vi "Update Control.vi"(8 "error in (no error)":errorcluster, 9 "Default Value Map":variant, 10 "Value":variant, 11 "Control Ref":refnum<vi>) -> (0 "error out":errorcluster, 1 "Label Text":string, 2 "Value":variant, 3 "Control Ref":refnum<vi>)   [LabVIEW 2019, in "User Interface.lvlib"]
doc: "Handles updating fill for knob and slide controls. Will also update output type as necessary (see note on block diagram)."
uses:
  User Interface.lvlib
  <vilib>/Utility/Data Type/NI_Data Type.lvlib
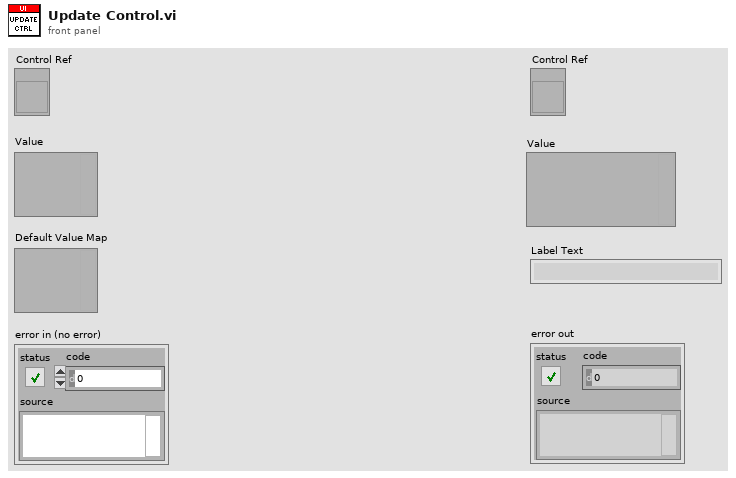
[diagram p1: front panel]
types:
  T1 = typedef "NI_Data Type.lvlib/Data Type.ctl" = enum8{"Invalid Type", "Void", "I8", "I16", "I32", "I64", "U8", "U16", "U32", "U64", "Single Float", "Double Float", "Extended Float", "Single Complex", "Double Complex", "Extended Complex", "Enum U8", "Enum U16", "Enum U32", "Enum U64", "Single Float With Unit", "Double Float With Unit", "Extended Float With Unit", "Single Complex with Unit", "Double Complex with Unit", "Extended Complex with Unit", "Boolean", "String", "Path", "Picture", "Tag", "Array", "Cluster", "Variant", "LV Variant", "Waveform", "Timestamp", "Digital Waveform", "Digital Data", "ExpressData", "Refnum", "External Data", "VI", "Poly VI", "LabVIEW Class Instance", "Fixed Point", "Set Collection", "Map Collection"}
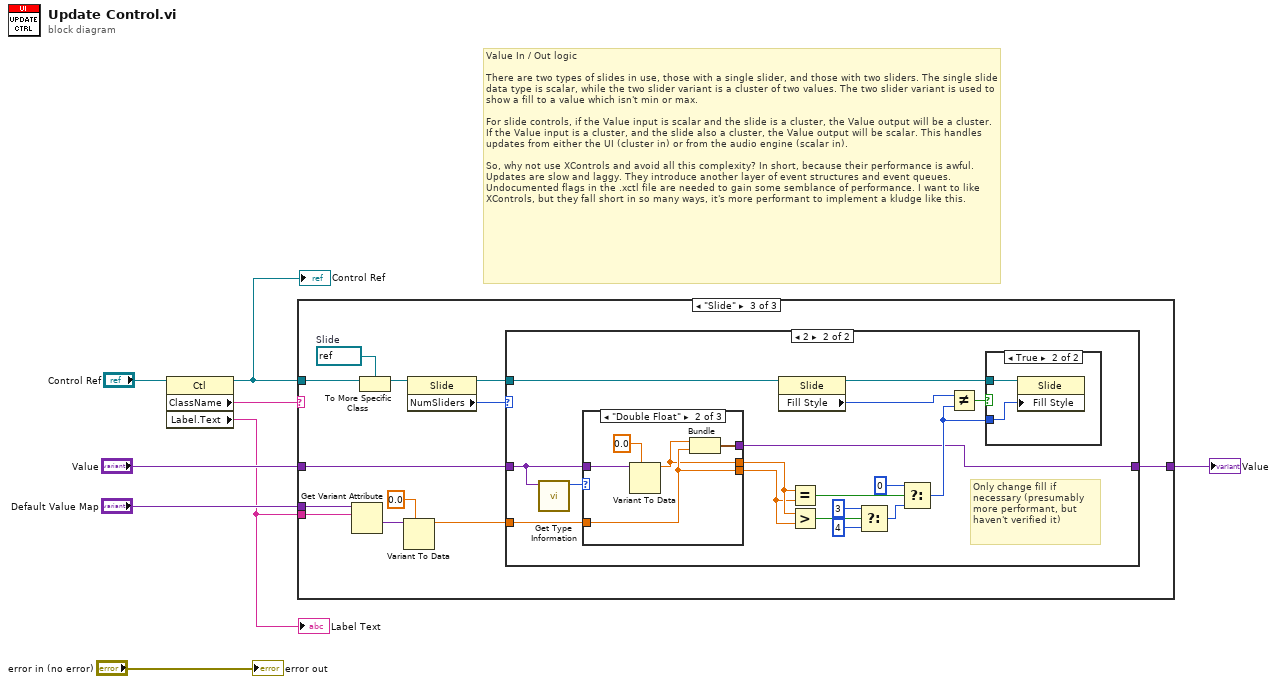
[diagram p0: block diagram]
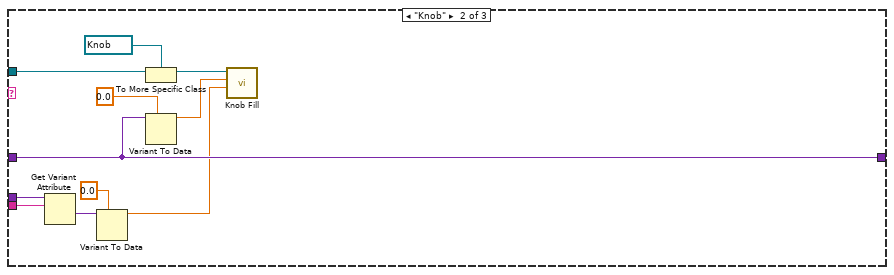
[diagram p3: hidden frame]
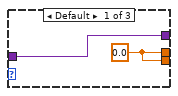
[diagram p5: hidden frame]
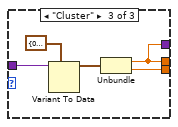
[diagram p6: hidden frame]
diagram:
  # "Value In / Out logic\n\nThere are two types of slides in use, those with a single slider, and those with two sliders. The single slide data type is scalar, while the two slider variant is a cluster of two values. The two slider variant is used to show a fill to a value which isn't min or max.\n\nFor slide controls, if the Value input is scalar and the slide is a cluster, the Value output will be a cluster. If the Value input is a cluster, and the slide also a cluster, the Value output will be scalar. This handles updates from either the UI (cluster in) or from the audio engine (scalar in).\n\nSo, why not use XControls and avoid all this complexity? In short, because their performance is awful. Updates are slow and laggy. They introduce another layer of event structures and event queues. Undocumented flags in the .xctl file are needed to gain some semblance of performance. I want to like XControls, but they fall short in so many ways, it's more performant to implement a kludge like this."
  n1 = property class="Ctl"(reference="Control Ref") -> (reference out=w4:refnum<vi>, "ClassName"=w7:string, "Label.Text"=w1:string)  [unwired: 1 in, 1 out]
  "Control Ref" <- w4
  "Label Text" <- w1
  n2 = case shown="\"Slide\"" w7 {
    tunnel: w4 -> [_ w17 w29]
    tunnel: "Value" -> [w9 w15 w32]
    tunnel: [w9 w15 w31] -> w5
    tunnel: w1 -> [_ w10 w23]
    tunnel: "Default Value Map" -> [_ w13 w24]
    frame Default {
    }
    frame "Knob" {
      n3 = Get Variant Attribute(Variant=w13, name=w10) -> (value=w11:variant)  [unwired: 2 in, 3 out]
      n4 = Variant To Data(type=0.0 ("y"), Variant=w11) -> (data=w12:dbl)  [unwired: 1 in, 1 out]
      n5 = To More Specific Class(target class=refnum<vi> refnum ("Knob Ref"), reference=w17) -> (specific class reference=w18:refnum<vi>)  [unwired: 1 in, 1 out]
      n6 = Variant To Data(type=0.0 ("y"), Variant=w15) -> (data=w16:dbl)  [unwired: 1 in, 1 out]
      n7 = call "Knob Fill.vi"("Default Value"=w12, "Value"=w16, "Knob Ref"=w18) -> ()  [unwired: 9 in]
    }
    frame "Slide" {
      w30 = refnum<vi> refnum  # Slide
      n8 = Get Variant Attribute(Variant=w24, name=w23) -> (value=w25:variant)  [unwired: 2 in, 3 out]
      n9 = To More Specific Class(target class=w30, reference=w29) -> (specific class reference=w28:refnum<vi>)  [unwired: 1 in, 1 out]
      n10 = Variant To Data(type=0.0 ("y"), Variant=w25) -> (data=w22:dbl)  [unwired: 1 in, 1 out]
      n11 = property class="Slide"(reference=w28) -> (reference out=w27:refnum<vi>, "NumSliders"=w21:i32)  [unwired: 1 in, 1 out]
      n12 = case shown="2" w21 {
        tunnel: w32 -> [w33 w37]
        tunnel: [w33 w34] -> w31
        tunnel: w27 -> [_ w38]
        tunnel: w22 -> [_ w35]
        frame Default {
        }
        frame 2 {
          # "Only change fill if necessary (presumably more performant, but haven't verified it)"
          n13 = call <vilib>:"Get Type Information.vi"("variant"=w37) -> ("type"=w36:T1)  [unwired: 6 in, 4 out]
          n14 = case shown="\"Double Float\"" w36 {
            tunnel: [w51 w54 w58] -> w47
            tunnel: [w51 w55 w60] -> w46
            tunnel: w37 -> [w52 w56 w59]
            tunnel: w35 -> [_ w55 _]
            tunnel: [w52 w53 w58] -> w34
            frame Default {
              w51 = 0.0 ("y")
            }
            frame "Double Float" {
              n15 = Variant To Data(type=0.0 ("y"), Variant=w56) -> (data=w54:dbl)  [unwired: 1 in, 1 out]
              n16 = Bundle("y"=w54, "y"=w55) -> (w53:cluster{"y":dbl, "y":dbl})  [unwired: 1 in]
            }
            frame "Cluster" {
              n17 = Variant To Data(type=cluster{dbl, dbl} {0.0, 0.0}, Variant=w59) -> (data=w61:cluster{dbl, dbl})  [unwired: 1 in, 1 out]
              n18 = Unbundle(w61) -> (w58:dbl, w60:dbl)
            }
          }
          n19 = property class="Slide"(reference=w38) -> (reference out=w49:refnum<vi>, "Fill Style"=w50:i32)  [unwired: 1 in, 1 out]
          n20 = Equal?(x=w47, y=w46) -> (x = y?=w45:bool)
          n21 = Greater?(x=w47, y=w46) -> (0:w43:bool)
          n22 = Select(t=3 ("Active Slider"), s=w43, f=4 ("Active Slider")) -> (s? t:f=w42:i32)
          n23 = Select(t=0 ("Active Slider"), s=w45, f=w42) -> (s? t:f=w41:i32)
          n24 = Not Equal?(x=w50, y=w41) -> (x != y?=w48:bool)
          n25 = case shown="True" w48 {
            tunnel: w49 -> [_ w64]
            tunnel: w41 -> [_ w63]
            frame False {
            }
            frame True {
              n26 = property class="Slide"(reference=w64, "Fill Style"=w63) -> ()  [unwired: 1 in, 2 out]
            }
          }
        }
      }
    }
  }
  "Value" <- w5
  "error out" <- "error in (no error)"
